vi "Export Routing and Faulting Custom Device.vi"(8 "error in":errorcluster, 9 "operation":T1(ring)=enum."replace or create with confirmation", 10 "datalog path (use dialog)":path, 11 "routing and faulting custom device in":T2 format="%.0x") -> (0 "error out":errorcluster, 3 "routing and faulting custom device out":T2 format="%.0x")   [LabVIEW 2020, in "Routing and Faulting Scripting.lvlib"]
doc: "Saves the configuration for the Routing and Faulting custom device as a datalog file. Import the datalog file by using <b>Import Routing and Faulting Custom Device.vi</b>."
uses:
  Routing and Faulting Scripting.lvlib
  <vilib>/NI VeriStand/Custom Device API/Custom Device Item Ref.ctl
  Dependencies.llb/Routing_and_Faulting_Scripting_Dependencies_ImportExport.lvlib
  <vilib>/NI VeriStand/Custom Device API/Custom Device API.lvlib
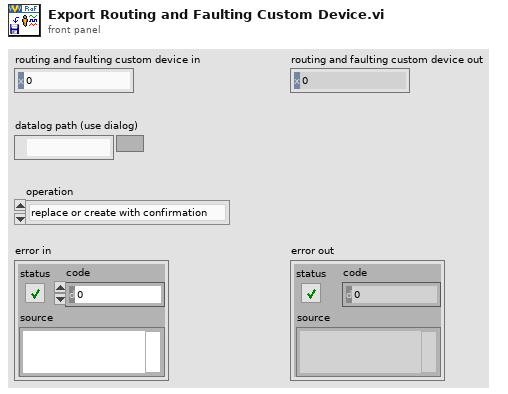
[diagram p1: front panel]
types:
  T1 = enum16{"open", "replace", "create", "open or create", "replace or create", "replace or create with confirmation"}
  T2 = typedef "Custom Device API.lvlib/Custom Device Item Ref.ctl" = u64
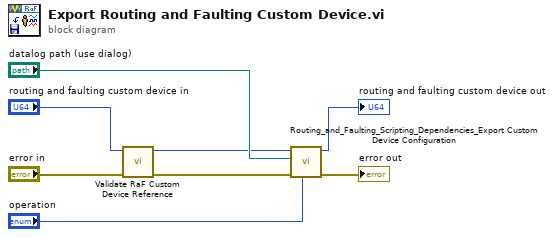
[diagram p0: block diagram]
diagram:
  n1 = call "Validate RaF Custom Device Reference.vi"("error in"="error in", "routing and faulting in"="routing and faulting custom device in") -> ("error out"=w3:errorcluster, "routing and faulting out"=w1:T2)  [unwired: 8 in]
  n2 = call "Routing_and_Faulting_Scripting_Dependencies_Export Custom Device Configuration.vi"("operation"="operation", "error in (no error)"=w3, "Path"="datalog path (use dialog)", "ID"=w1) -> ("error out"=→"error out":errorcluster, "ID out"=→"routing and faulting custom device out":u64)  [unwired: 6 in]
